vi "Store Delay.vi"(8 "Levels":u8, 9 "Data In":fxp<+/-,8,8>) -> (1 "Data Out":fxp<+/-,8,8>)   [LabVIEW 2015]
doc: "Chains up to 16 Feedback Nodes, all configured with a 512 Delay value, applying echo effect to the input signal."
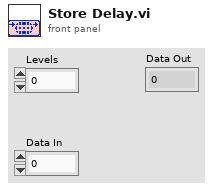
[diagram p1: front panel]
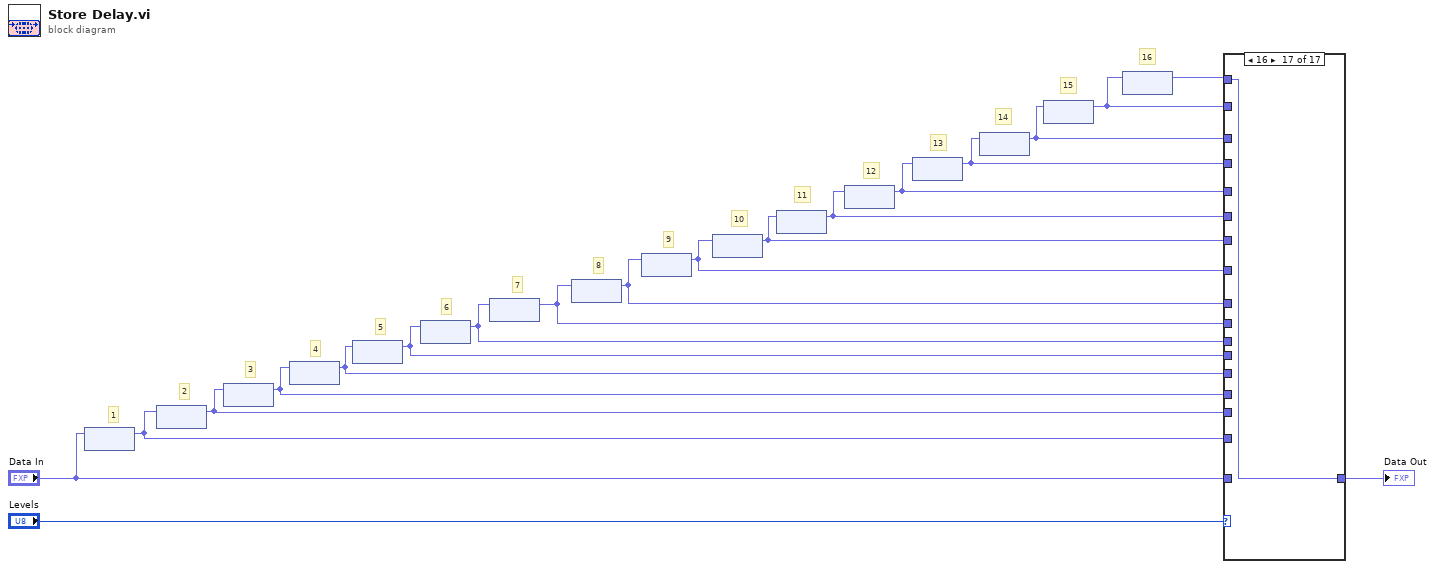
[diagram p0: block diagram]
diagram:
  # "16"
  # "15"
  # "14"
  # "13"
  # "12"
  # "11"
  # "10"
  # "9"
  # "8"
  # "7"
  # "6"
  # "5"
  # "4"
  # "3"
  # "2"
  # "1"
  n1 = feedback #1() -> (w17:fxp<+/-,8,8>)  [unwired: 1 in]
  n2 = feedback-in #1("Data In") -> ()
  n3 = feedback #2() -> (w16:fxp<+/-,8,8>)  [unwired: 1 in]
  n4 = feedback-in #2(w17) -> ()
  n5 = feedback #3() -> (w15:fxp<+/-,8,8>)  [unwired: 1 in]
  n6 = feedback-in #3(w16) -> ()
  n7 = feedback #4() -> (w14:fxp<+/-,8,8>)  [unwired: 1 in]
  n8 = feedback-in #4(w15) -> ()
  n9 = feedback #5() -> (w13:fxp<+/-,8,8>)  [unwired: 1 in]
  n10 = feedback-in #5(w14) -> ()
  n11 = feedback #6() -> (w12:fxp<+/-,8,8>)  [unwired: 1 in]
  n12 = feedback-in #6(w13) -> ()
  n13 = feedback #7() -> (w11:fxp<+/-,8,8>)  [unwired: 1 in]
  n14 = feedback-in #7(w12) -> ()
  n15 = feedback #8() -> (w9:fxp<+/-,8,8>)  [unwired: 1 in]
  n16 = feedback-in #8(w11) -> ()
  n17 = feedback #9() -> (w8:fxp<+/-,8,8>)  [unwired: 1 in]
  n18 = feedback-in #9(w9) -> ()
  n19 = feedback #10() -> (w7:fxp<+/-,8,8>)  [unwired: 1 in]
  n20 = feedback-in #10(w8) -> ()
  n21 = feedback #11() -> (w6:fxp<+/-,8,8>)  [unwired: 1 in]
  n22 = feedback-in #11(w7) -> ()
  n23 = feedback #12() -> (w5:fxp<+/-,8,8>)  [unwired: 1 in]
  n24 = feedback-in #12(w6) -> ()
  n25 = feedback #13() -> (w4:fxp<+/-,8,8>)  [unwired: 1 in]
  n26 = feedback-in #13(w5) -> ()
  n27 = feedback #14() -> (w3:fxp<+/-,8,8>)  [unwired: 1 in]
  n28 = feedback-in #14(w4) -> ()
  n29 = feedback #15() -> (w2:fxp<+/-,8,8>)  [unwired: 1 in]
  n30 = feedback-in #15(w3) -> ()
  n31 = feedback #16() -> (w1:fxp<+/-,8,8>)  [unwired: 1 in]
  n32 = feedback-in #16(w2) -> ()
  n33 = case shown="16" "Levels" {
    tunnel: "Data In" -> [w20 _ _ _ _ _ _ _ _ _ _ _ _ _ _ _ _]
    tunnel: w17 -> [_ w21 _ _ _ _ _ _ _ _ _ _ _ _ _ _ _]
    tunnel: w16 -> [_ _ w22 _ _ _ _ _ _ _ _ _ _ _ _ _ _]
    tunnel: w15 -> [_ _ _ w23 _ _ _ _ _ _ _ _ _ _ _ _ _]
    tunnel: w14 -> [_ _ _ _ w24 _ _ _ _ _ _ _ _ _ _ _ _]
    tunnel: w13 -> [_ _ _ _ _ w25 _ _ _ _ _ _ _ _ _ _ _]
    tunnel: w12 -> [_ _ _ _ _ _ w26 _ _ _ _ _ _ _ _ _ _]
    tunnel: w11 -> [_ _ _ _ _ _ _ w27 _ _ _ _ _ _ _ _ _]
    tunnel: w9 -> [_ _ _ _ _ _ _ _ w28 _ _ _ _ _ _ _ _]
    tunnel: [w20 w21 w22 w23 w24 w25 w26 w27 w28 w29 w30 w31 w32 w33 w34 w35 w36] -> w10
    tunnel: w8 -> [_ _ _ _ _ _ _ _ _ w29 _ _ _ _ _ _ _]
    tunnel: w7 -> [_ _ _ _ _ _ _ _ _ _ w30 _ _ _ _ _ _]
    tunnel: w6 -> [_ _ _ _ _ _ _ _ _ _ _ w31 _ _ _ _ _]
    tunnel: w5 -> [_ _ _ _ _ _ _ _ _ _ _ _ w32 _ _ _ _]
    tunnel: w4 -> [_ _ _ _ _ _ _ _ _ _ _ _ _ w33 _ _ _]
    tunnel: w3 -> [_ _ _ _ _ _ _ _ _ _ _ _ _ _ w34 _ _]
    tunnel: w2 -> [_ _ _ _ _ _ _ _ _ _ _ _ _ _ _ w35 _]
    tunnel: w1 -> [_ _ _ _ _ _ _ _ _ _ _ _ _ _ _ _ w36]
    frame 0, Default {
    }
    frame 1 {
    }
    frame 2 {
    }
    frame 3 {
    }
    frame 4 {
    }
    frame 5 {
    }
    frame 6 {
    }
    frame 7 {
    }
    frame 8 {
    }
    frame 9 {
    }
    frame 10 {
    }
    frame 11 {
    }
    frame 12 {
    }
    frame 13 {
    }
    frame 14 {
    }
    frame 15 {
    }
    frame 16 {
    }
  }
  "Data Out" <- w10
